vi "Save VI File Without Diagram.vi"(8 "error in (no error)":errorcluster, 10 "Folder Path(For Saved)":path, 11 "VI File Path(Need Save)":path) -> (0 "error out":errorcluster, 3 "Result":bool)   [LabVIEW 2013]
doc: "Save the *.vi file without diagram."
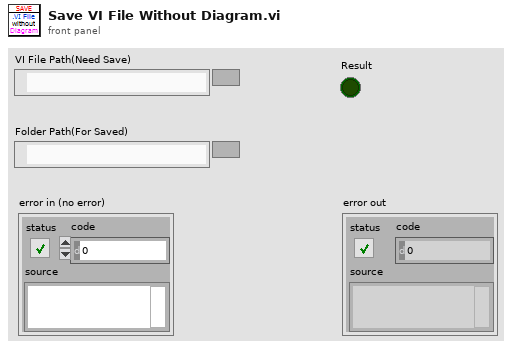
[diagram p1: front panel]
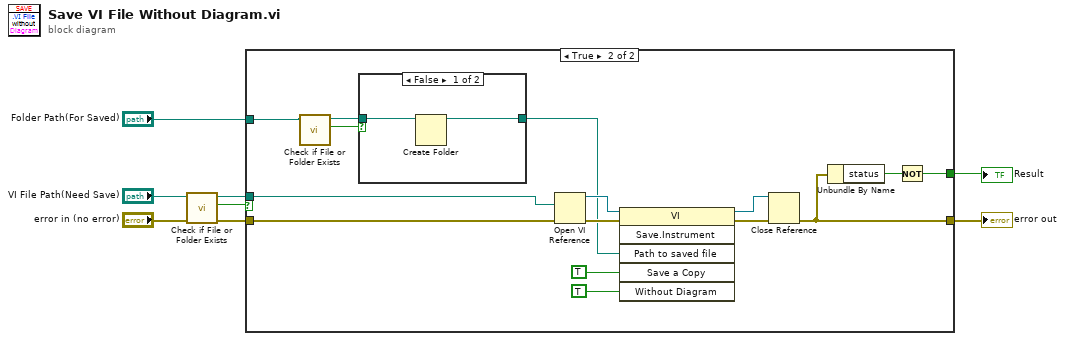
[diagram p0: block diagram]
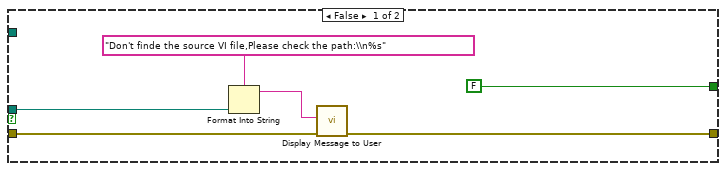
[diagram p2: hidden frame]
diagram:
  n1 = call <vilib>:"Check if File or Folder Exists.vi"("error in (no error)"="error in (no error)", "path"="VI File Path(Need Save)") -> ("error out"=w4:errorcluster, "file or folder exists?"=w2:bool, "dup path"=w3:path)  [unwired: 7 in]
  n2 = case shown="True" w2 {
    tunnel: "Folder Path(For Saved)" -> [_ w21]
    tunnel: [w13 w20] -> w7
    tunnel: w4 -> [w14 w23]
    tunnel: w3 -> [w10 w22]
    tunnel: [FALSE w18] -> w1
    frame False {
      n3 = Format Into String(format string="Don't finde the source VI file,Please check the path:\\n%s" ("Message"), w10) -> (resulting string=w9:string)  [unwired: 2 in, 1 out]
      n4 = call "Display Message to User"("error in (no error)"=w14, "Message"=w9) -> ("error out"=w13:errorcluster)  [unwired: 8 in, 1 out]
    }
    frame True {
      n5 = call <vilib>:"Check if File or Folder Exists.vi"("path"=w21) -> ("file or folder exists?"=w17:bool, "dup path"=w15:path)  [unwired: 8 in, 1 out]
      n6 = case shown="False" w17 {
        tunnel: [w30 w32] -> w16
        tunnel: w15 -> [w31 w32]
        frame False {
          n7 = Create Folder(path (use dialog)=w31) -> (created path=w30:path)  [unwired: 2 in, 2 out]
        }
        frame True {
        }
      }
      n8 = Open VI Reference(vi path=w22, error in (no error)=w23) -> (vi reference=w28:refnum<vi>, error out=w29:errorcluster)  [unwired: 4 in]
      n9 = invoke class="VI" method="Save.Instrument"(reference=w28, error in=w29, "Path to saved file"=w16, "Save a Copy"=TRUE, "Without Diagram"=TRUE) -> (reference out=w24:refnum<vi>, error out=w25:errorcluster)  [unwired: 1 in, 4 out]
      n10 = Close Reference(reference=w24, error in (no error)=w25) -> (error out=w20:errorcluster)
      n11 = Unbundle By Name(w20) -> ("status"=w19:bool)
      n12 = Not(x=w19) -> (.not. x?=w18:bool)
    }
  }
  "error out" <- w7
  "Result" <- w1
